vi "Joystick Tracker R2.vi"() -> ()   [LabVIEW 2014]
uses:
  <vilib>/MakerHub/LINX/Public/Peripherals/Analog/Analog Read N Chans.vi
  <vilib>/MakerHub/LINX/Private/Local IO/LinxAnalogRead.vi
  <vilib>/MakerHub/LINX/Public/Utilities/Check Channel.vi
  <vilib>/MakerHub/LINX/Public/Utilities/Open Serial.vi
  <vilib>/MakerHub/LINX/Private/Utilties/Generate Error.vi
  <vilib>/MakerHub/LINX/LMH-LINX.lvlib
panel:
  out "Click Value":cluster{dbl[], dbl[]} {"?" format="%.2g"; "?" format="%.2g"}
  out "String":string
  in  "V_2 Trim":dbl(c297)=9.281437125748258e-05
  in  "V_1 Trim":dbl(c297)=-0.0017611464968152863
  out "Voltage Outputs":dbl[](array[numeric]) format="%_4g"
  out "Joystick Plot":cluster{dbl[], dbl[]}(graph)
  in  "AI Channel(s)":u8[](array[numeric])=[0, 1, 2]
  in  "Stop Button":bool
  out "Loop Rate (Hz)":u32
  in  "Serial Port":refnum<visa-resource-name>="COM9"
  # "Joystick Plot"
  # "Setup"
  # "V_0"
  # "V_1"
  # "V_2"
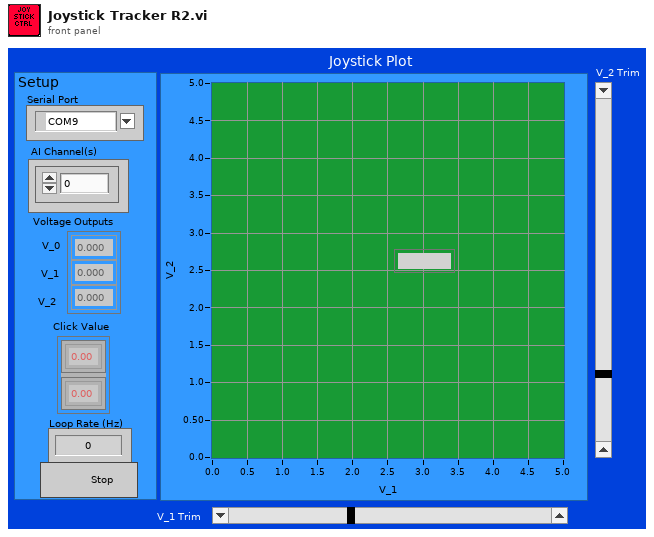
[diagram p1: front panel]
types:
  T1 = typedef "LMH-LINX.lvlib/LINX Ref.ctl" = cluster{"IO":T2, "Interface":T3, "LINX Device Config":T4}
  T2 = typedef "LMH-LINX.lvlib/Platform.ctl" = enum16{"Remote", "Local"}
  T3 = typedef "LMH-LINX.lvlib/Interface.ctl" = enum16{"Serial", "TCP"}
  T4 = typedef "LMH-LINX.lvlib/Device.lvlib/LINX Device Config.ctl" = cluster{"Interface":T3, "COM Port":refnum<visa-resource-name>, "TCP Configuration":T5, "Device Family":u8, "Device ID":u8, "Device Name":string, "TCP Ref":refnum<k5>, "Channels":T6}
  T5 = typedef "LMH-LINX.lvlib/Device.lvlib/TCP Config.ctl" = cluster{"IP Address":string, "Port":u16}
  T6 = typedef "LMH-LINX.lvlib/Channels.ctl" = cluster{"DI":u8[], "DO":u8[], "AI":u8[], "AO":u8[], "PWM":u8[], "QE":u8[], "UART":u8[], "I2C 2":u8[], "SPI":u8[], "CAN":u8[], "Servo":u8[], "AI Ref (V)":dbl, "AI Resolution (Bits)":u8, "AO Ref (V)":dbl, "AO Resolution (Bits)":u8}
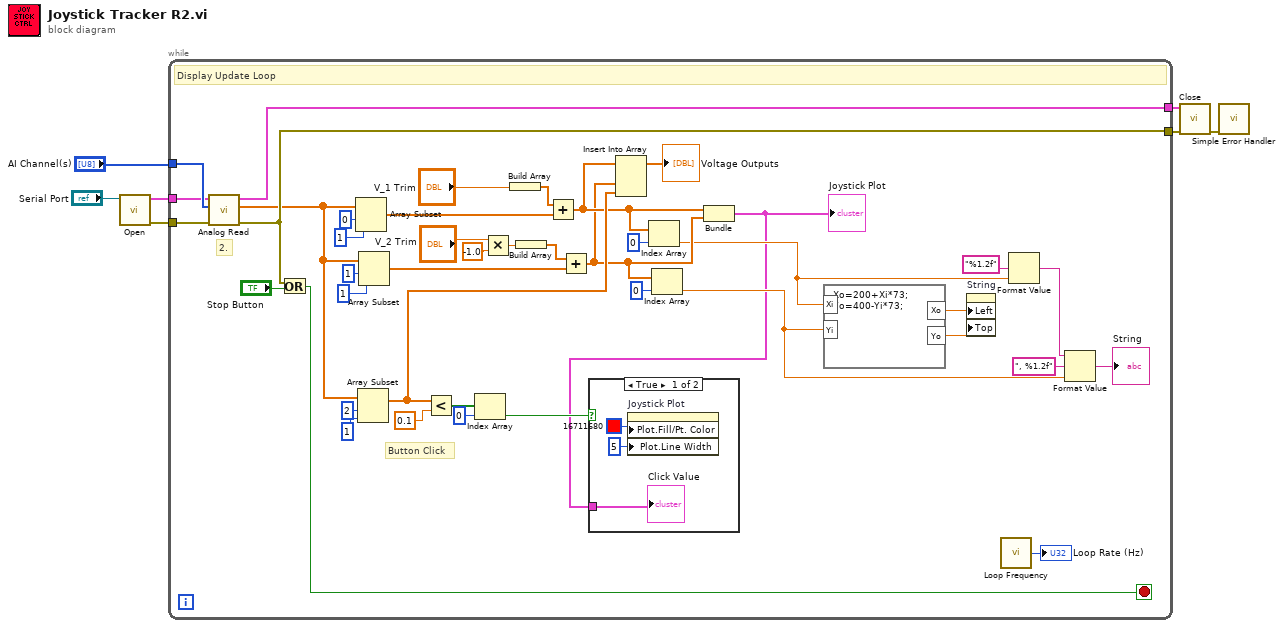
[diagram p0: block diagram]
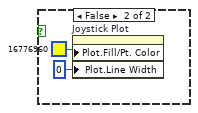
[diagram p2: hidden frame]
diagram:
  n1 = call-poly <vilib>:"Open.vi"("Serial Port"="Serial Port") -> ("Error Out"=w1:errorcluster, "LINX Resource"=w2:T1)  [unwired: 8 in, 1 out]
  n2 = while {
    tunnel: "AI Channel(s)" -> [w47]
    tunnel: [w46] -> w5
    tunnel: [w45] -> w4
    tunnel: w2 -> [w44]
    tunnel: w1 -> [w43]
    stop <- w36 stop-if-true
    # "Button Click"
    # "2."
    # "Display Update Loop"
    n3 = call-poly <vilib>:"Analog Read.vi"("Error In"=w43, "AI Channel(s)"=w47, "LINX Resource"=w44) -> ("Error Out"=w45:errorcluster, "Voltages"=w32:dbl[], "LINX Resource"=w46:T1)  [unwired: 5 in, 1 out]
    n4 = Or(x=w45, y="Stop Button") -> (x .or. y?=w36:bool)
    n5 = Array Subset(array=w32, index=0, length=1) -> (w30:dbl[])
    n6 = Array Subset(array=w32, index=2, length=1) -> (w27:dbl[])
    n7 = Array Subset(array=w32, index=1, length=1) -> (w25:dbl[])
    n8 = Less?(x=w27, y=0.1) -> (x < y?=w40:bool[])
    n9 = Index Array(array=w40, index=0) -> (element=w9:bool)
    n10 = Multiply(x="V_2 Trim", y=-1.0) -> (x*y=w22:dbl)
    n11 = Build Array("V_1 Trim") -> (w29:dbl[])
    n12 = Build Array(w22) -> (w26:dbl[])
    n13 = Add(x=w29, y=w30) -> (x+y=w21:dbl[])
    n14 = Add(x=w26, y=w25) -> (x+y=w20:dbl[])
    n15 = Insert Into Array(array=w21, new element #1=w20, new element #2=w27) -> (→"Voltage Outputs":dbl[])  [unwired: 1 in]
    n16 = Index Array(array=w21, index=0) -> (element=w15:dbl)
    n17 = Index Array(array=w20, index=0) -> (element=w13:dbl)
    n18 = Bundle(w21, w20) -> (w8:cluster{dbl[], dbl[]})  [unwired: 1 in]
    "Joystick Plot" <- w8
    n19 = case shown="True" w9 {
      tunnel: w8 -> [w50 _]
      frame True {
        n20 = property on="Joystick Plot" class="XYGraph (strict)"("Plot.Fill/Pt. Color"=u32 16711680, "Plot.Line Width"=u8 5) -> ()  [unwired: 2 in, 2 out]
        "Click Value" <- w50
      }
      frame False {
        n21 = property on="Joystick Plot" class="XYGraph (strict)"("Plot.Fill/Pt. Color"=u32 16776960, "Plot.Line Width"=u8 0) -> ()  [unwired: 2 in, 2 out]
      }
    }
    n22 = formula code="Xo=200+Xi*73;\nYo=400-Yi*73;"("Xi"=w15, "Yi"=w13) -> ("Xo"=w17:dbl, "Yo"=w16:dbl)
    n23 = property on="String" class="Str"("Left"=w17, "Top"=w16) -> ()  [unwired: 2 in, 2 out]
    n24 = call <vilib>:"Loop Frequency.vi"() -> ("Loop Rate (Hz)"=→"Loop Rate (Hz)":u32)
    n25 = Format Value(format string="%1.2f", value (0)=w15) -> (output string=w11:string)  [unwired: 1 in]
    n26 = Format Value(string ("")=w11, format string=", %1.2f", value (0)=w13) -> (output string=→"String":string)
  }
  n27 = call <vilib>:"Close.vi"("Error In"=w4, "LINX Resource"=w5) -> ("Error Out"=w6:errorcluster)  [unwired: 9 in]
  n28 = call <vilib>:"Simple Error Handler.vi"("error in (no error)"=w6) -> ()  [unwired: 4 in, 5 out]
